vi "Auxiliary Association (Set).vi"(6 "ISOBUS address":T2=-1 caption="ISOBUS address (-1)", 8 "error in":errorcluster, 10 "Auxiliary UID":string, 11 "Mercury Reference In":T4) -> (0 "error out":errorcluster, 2 "Response":T1, 3 "Mercury Reference Out":T4, 4 "Valid?":T3)   [LabVIEW 2013, in "Mercury iXX.lvlib" / "Control Loop.lvlib"]
doc: "Set the UID of the associated auxiliary board to the control loop.\nSet value to 0 to unset association."
uses:
  Control Loop.lvlib
  Mercury iXX.lvlib
  Private/Controls/Command Verbs.ctl
  Controls/Is Valid LED.ctl
  Controls/Response String.ctl
  Controls/Comms Transport Layer.ctl
  Private/Controls/Query Dynamic Reference.ctl
  Controls/Mercury Reference.ctl
  Controls/ISOBus Address.ctl
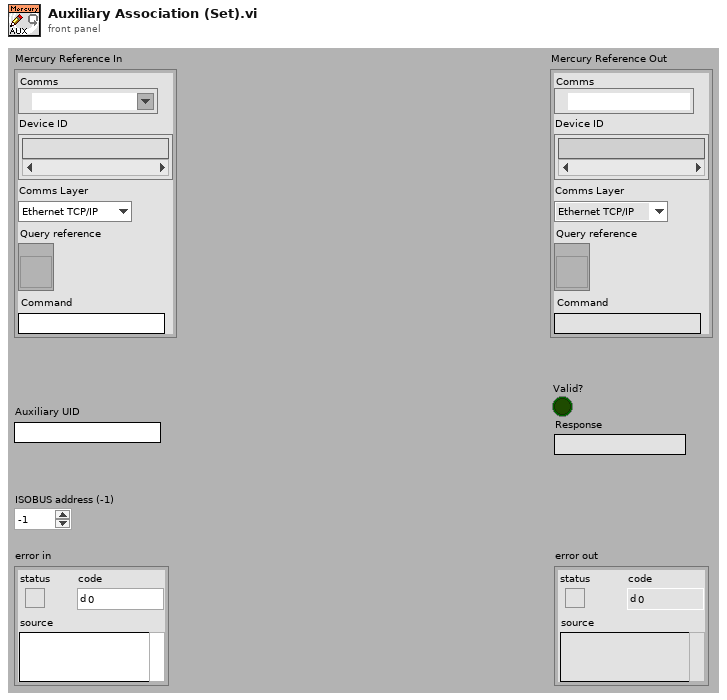
[diagram p1: front panel]
types:
  T1 = typedef "Mercury iXX.lvlib/Response String.ctl" = string
  T2 = typedef "Mercury iXX.lvlib/ISOBus Address.ctl" = i32
  T3 = typedef "Mercury iXX.lvlib/Is Valid LED.ctl" = bool
  T4 = typedef "Mercury iXX.lvlib/Mercury Reference.ctl" = cluster{"Comms":refnum<visa-resource-name>, "Device ID":string[], "Comms Layer":T5, "Command":string, "Query reference":T6}
  T5 = typedef "Mercury iXX.lvlib/Comms Transport Layer.ctl" = enum16{"Ethernet TCP/IP", "USB", "ISOBus - RS-232", "GPIB"}
  T6 = typedef "Mercury iXX.lvlib/Query Dynamic Reference.ctl" = refnum<vi>
  T7 = typedef "Mercury iXX.lvlib/Command Verbs.ctl" = string
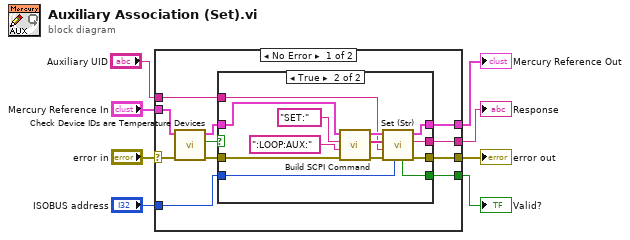
[diagram p0: block diagram]
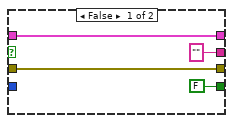
[diagram p2: hidden frame]
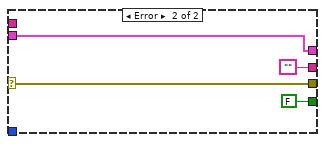
[diagram p3: hidden frame]
diagram:
  n1 = case shown="No Error" "error in" {
    selector: "error in" -> [w16 w39]
    tunnel: "Mercury Reference In" -> [w13 w40]
    tunnel: [w19 w40] -> w5
    tunnel: [w18 w39] -> w8
    tunnel: [w9 ""] -> w1
    tunnel: [w10 FALSE ("Valid?")] -> w2
    tunnel: "ISOBUS address" -> [w12 _]
    tunnel: "Auxiliary UID" -> [w11 _]
    frame No Error {
      n2 = call "Check Device IDs are Temperature Devices.vi"("error in"=w16, "Mercury Reference In"=w13) -> ("error out"=w15:errorcluster, "Valid?"=w17:bool, "Mercury Reference Out"=w14:T4)  [unwired: 7 out]
      n3 = case shown="True" w17 {
        tunnel: w15 -> [w22 w29]
        tunnel: w14 -> [w23 w28]
        tunnel: [w23 w31] -> w19
        tunnel: [w22 w30] -> w18
        tunnel: w12 -> [_ w27]
        tunnel: w11 -> [_ w26]
        tunnel: [T3 FALSE ("Valid?") w25] -> w10
        tunnel: [T1 "" ("Response") w24] -> w9
        frame False {
        }
        frame True {
          n4 = call "Build SCPI Command.vi"("error in"=w29, "Noun(s)"=":LOOP:AUX:" ("Command"), "Verb"=T7 "SET:", "Mercury Reference In"=w28) -> ("error out"=w35:errorcluster, "SCPI Message(s)"=w34:string[], "Mercury Reference Out"=w33:T4)  [unwired: 5 out]
          n5 = call "Set (Str).vi"("ISOBUS address"=w27, "error in"=w35, "Command Value (Str)"=w26, "SCPI Message(s)"=w34, "Mercury Reference In"=w33) -> ("error out"=w30:errorcluster, "Response"=w24:T1, "Mercury Reference Out"=w31:T4, "Valid?"=w25:T3)  [unwired: 3 out]
        }
      }
    }
    frame Error {
    }
  }
  "Mercury Reference Out" <- w5
  "error out" <- w8
  "Valid?" <- w2
  "Response" <- w1
